vi "Post-Build Action.vi"(5 "Files Generated by Build":path[](array[path]), 6 "Top Level/Always Included VIs":path[](array[path]), 7 "Destination Path":path, 8 "error in (no error)":errorcluster, 9 "Target Name":string, 10 "Build Specification Name":string, 11 "Project Path":path) -> (0 "error out":errorcluster)   [LabVIEW 2020]
uses:
  <vilib>/Utility/error.llb/Error Cluster From Error Code.vi
  <vilib>/regexp/Match Regular Expression.xnode
  <vilib>/ErrorRing/Error Ring.xnode
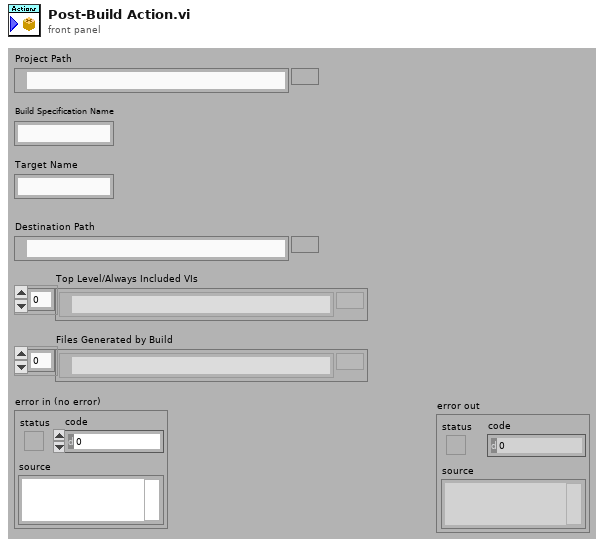
[diagram p1: front panel]
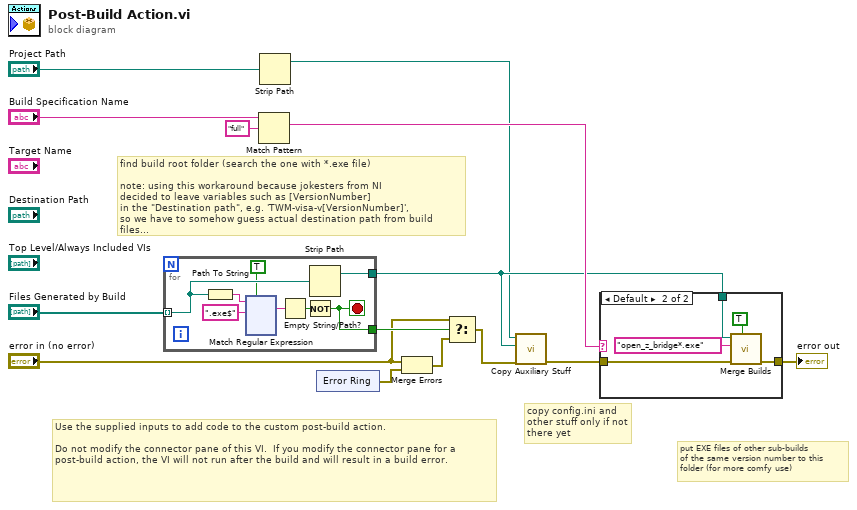
[diagram p0: block diagram]
diagram:
  # "copy config.ini and\nother stuff only if not\nthere yet"
  # "put EXE files of other sub-builds\nof the same version number to this\nfolder (for more comfy use)"
  # "find build root folder (search the one with *.exe file)\n\nnote: using this workaround because jokesters from NI\ndecided to leave variables such as [VersionNumber]\nin the \"Destination path\", e.g. 'TWM-visa-v[VersionNumber]',\nso we have to somehow guess actual destination path from build files..."
  # "Use the supplied inputs to add code to the custom post-build action.\n\nDo not modify the connector pane of this VI.  If you modify the connector pane for a post-build action, the VI will not run after the build and will result in a build error."
  n1 = for {
    tunnel: "Files Generated by Build" -> [w19] mode=indexing
    tunnel: [w18] -> w3
    tunnel: [w16] -> w12
    stop <- w16 stop-if-true
    n2 = Path To String(path=w19) -> (string=w21:string)
    n3 = xnode "Match Regular Expression"("input string"=w21, "regular expression"=".exe$", "ignore case? (F)"=TRUE) -> ("whole match"=w20:string)  [unwired: 3 in, 4 out]
    n4 = Empty String/Path?(string/path=w20) -> (empty?=w17:bool)
    n5 = Not(x=w17) -> (.not. x?=w16:bool)
    n6 = Strip Path(path=w19) -> (stripped path=w18:path)  [unwired: 1 out]
  }
  n7 = Match Pattern(string="Build Specification Name", regular expression="full") -> (match substring=w5:string)  [unwired: 1 in, 3 out]
  n8 = Strip Path(path="Project Path") -> (stripped path=w1:path)  [unwired: 1 out]
  n9 = xnode "Error Ring"() -> ("error out"=w13:errorcluster)
  n10 = Merge Errors("error in (no error)", w13) -> (w11:errorcluster)
  n11 = Select(t="error in (no error)", s=w12, f=w11) -> (s? t:f=w4:errorcluster)
  n12 = call "Copy Auxiliary Stuff.vi"("error in"=w4, "Build Destination Folder Path"=w3, "lvProject folder path"=w1) -> ("error out"=w2:errorcluster)  [unwired: 8 in]
  n13 = case shown="Default" w5 {
    tunnel: w2 -> [w137 w142]
    tunnel: w3 -> [_ w141]
    tunnel: [w137 w140] -> w8
    frame "" {
    }
    frame Default {
      n14 = call "Merge Builds.vi"("Offer remove other builds after merge? (False)"=TRUE, "error in"=w142, "wildcard serach key for exe file (e.g.: power?cal*.exe)"="open_z_bridge*.exe", "Destination Path"=w141) -> ("error out"=w140:errorcluster)  [unwired: 6 in, 1 out]
    }
  }
  "error out" <- w8
